vi "Set Server Internal UEs.vi"(10 "Server Internal UEs":T1, 11 "OOP Server in":refnum<class "Template Server.lvclass">) -> (3 "OOP Server out":refnum<class "Template Server.lvclass">)   [LabVIEW 2019, in "Template Server.lvlib" / "Template Server.lvclass"]
uses:
  Template Server.lvclass
  typeDefs/Server Internal UEs.ctl
  typeDefs/Server Internal Data.ctl
  Template Server.lvclass/Template Server.ctl
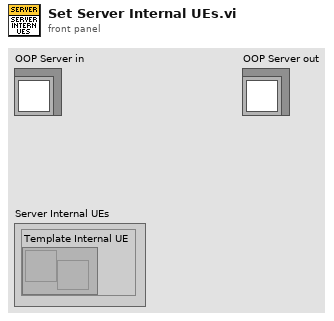
[diagram p1: front panel]
types:
  T1 = typedef "Template Server.lvlib/Template Server.lvclass/Server Internal UEs.ctl" = cluster{"Template Internal UE":refnum<user-event>}
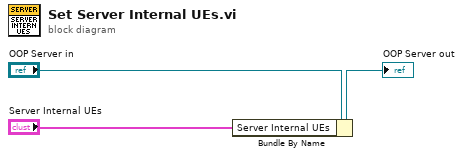
[diagram p0: block diagram]
diagram:
  n1 = Bundle By Name(cluster="OOP Server in", "Server Internal UEs"="Server Internal UEs") -> (→"OOP Server out":refnum<class "Template Server.lvclass">)
